vi "TagContainer-IsValid.vi"(8 "error in (no error)":errorcluster, 11 "TagContainer":T1) -> (0 "error out":errorcluster, 2 "valid TagContainer?":bool, 3 "TagContainer(dup)":T1)   [LabVIEW 2017, in "TagContainer.lvlib"]
uses:
  TagContainer.lvlib
  Typedef/TagContainer.ctl
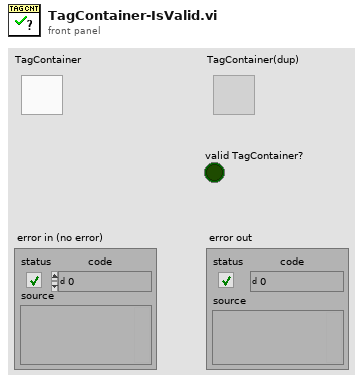
[diagram p1: front panel]
types:
  T1 = typedef "TagContainer.lvlib/TagContainer.ctl" = refnum<k1>
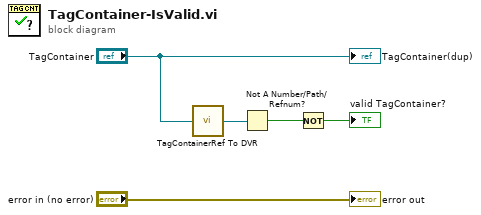
[diagram p0: block diagram]
diagram:
  n1 = call "TagContainerRef To DVR.vi"("TagContainer"="TagContainer") -> ("DVR"=w3:refnum<data-value>)
  n2 = Not A Number/Path/Refnum?(number/path/refnum=w3) -> (NaN/Path/Refnum?=w2:bool)
  n3 = Not(x=w2) -> (.not. x?=→"valid TagContainer?":bool)
  "error out" <- "error in (no error)"
  "TagContainer(dup)" <- "TagContainer"
